vi "ASDA-A2_Get Position Data.vi"(8 "error in":errorcluster, 11 "Buffer Data In":T1) -> (0 "error out":errorcluster, 2 "Position":cluster{"CN2 Encoder":i32, "CN5 Encoder":i32}, 3 "Buffer Data Out":T1)   [LabVIEW 2016]
uses:
  Data Def/ASDA-A2_Buffer Data.ctl
  Data Def/ASDA-A2_Read Register Data.ctl
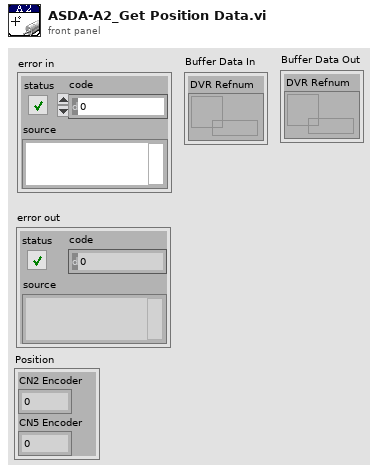
[diagram p1: front panel]
types:
  T1 = typedef "ASDA-A2_Buffer Data.ctl" = cluster{"DVR Refnum":refnum<data-value>}
  T2 = typedef "ASDA-A2_Read Register Data.ctl" = cluster{"Address":u16, "Count":u16, "Page":string, "Description":string}
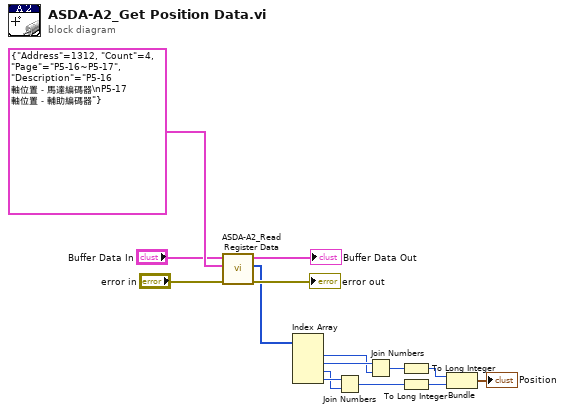
[diagram p0: block diagram]
diagram:
  n1 = call "ASDA-A2_Read Register Data.vi"("error in"="error in", "Read Register Data"=T2 {"Address"=1312, "Count"=4, "Page"="P5-16~P5-17", "Description"="P5-16 軸位置－馬達編碼器\nP5-17 軸位置－輔助編碼器"}, "Buffer Data In"="Buffer Data In") -> ("error out"=→"error out":errorcluster, "Data"=w10:u16[], "Buffer Data Out"=→"Buffer Data Out":T1)  [unwired: 6 in]
  n2 = Index Array(array=w10) -> (element #1=w8:u16, element #2=w9:u16, element #3=w6:u16, element #4=w7:u16)  [unwired: 4 in]
  n3 = Join Numbers(hi=w7, lo=w6) -> ((hi.lo)=w3:u32)
  n4 = Join Numbers(hi=w9, lo=w8) -> ((hi.lo)=w4:u32)
  n5 = To Long Integer(number=w4) -> (32bit integer=w1:i32)
  n6 = To Long Integer(number=w3) -> (32bit integer=w2:i32)
  n7 = Bundle(w1, w2) -> (→"Position":cluster{i32, i32})  [unwired: 1 in]
